vi "WaitButtonPress.vi"(8 "error in":errorcluster, 11 "GlobalDataRef":refnum<data-value>) -> (0 "error out":errorcluster, 1 "Timed Out":bool, 2 "Short=1, (Long=0)Press":bool, 3 "GlobalDataRef":refnum<data-value>)   [LabVIEW 2015]
uses:
  ProjectFiles/TypeDefs/GlobalData.ctl
  Telegram/Methods/TypeDefs/ReplyKeyboardMarkup.ctl
  <vilib>/Utility/error.llb/Error Cluster From Error Code.vi
  <vilib>/RVI Host/nirviSupport.llb/nirviErrorClusterFromErrorCode.vi
  <vilib>/rvi/errors/niLvFpgaAdjustHostInterfaceError.vi
  <vilib>/rvi/interface/nirviMethod/nirviMethod.xnode
  <vilib>/rvi/interface/nirviReadWriteControl/nirviReadWriteControl.xnode
  <vilib>/rvi/interface/nirviMethod/StockFPGA_InlinedMethodWaitForSingleIRQ.vi
  <vilib>/FPGAPlugInAG/Dynamic/niLvFpga_WaitOnIrq_Dynamic.vi
  <vilib>/FPGAPlugInAG/Dynamic/niLvFpga_AcknowledgeIrq_Dynamic.vi
  NiFpgaLv.dll
  <vilib>/rvi/interface/Simulation/niFpgaSimulationCallBeginRW.vi
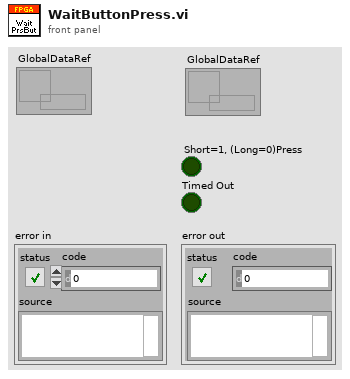
[diagram p1: front panel]
types:
  T1 = typedef "GlobalData.ctl" = cluster{"FPGA VI Ref":refnum<k20>, "Token":string, "ActiveChats":cluster{"ChatId":i32, "Type":string}[], "ActiveKeyboards":cluster{"Chat#":i32, "ReplyKeyboardMarkup":T2}[], "RefStringIn":refnum<vi>}
  T2 = typedef "ReplyKeyboardMarkup.ctl" = cluster{"keyboard":cluster{"text":string, "req_loc":bool}[][], "resize_keyboard":bool, "one_time_keyboard":bool, "selective":bool}
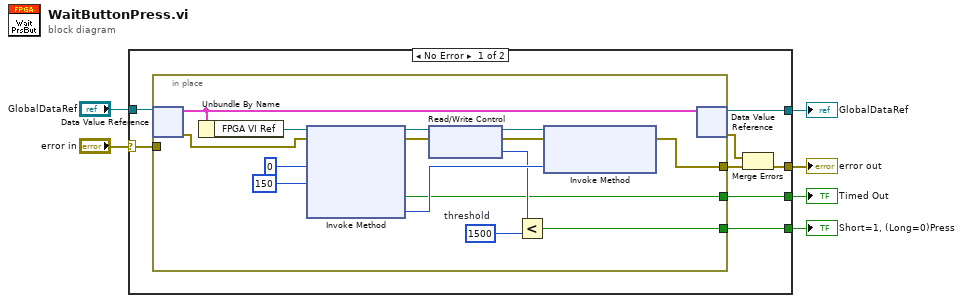
[diagram p0: block diagram]
diagram:
  n1 = case shown="No Error" "error in" {
    selector: "error in" -> [w13 w31]
    tunnel: "GlobalDataRef" -> [w14 w30]
    tunnel: [w12 _] -> w4
    tunnel: [w11 _] -> w3
    tunnel: [w7 w31] -> w2
    tunnel: [w10 w30] -> w1
    frame No Error {
      n2 = in-place {
        in-place-border: w13 -> [_]
        in-place-border: [w18] -> w9
        in-place-border: [w16] -> w12
        in-place-border: [w15] -> w11
        w20 = i16 1500  # threshold
        n3 = in-place-dvr #1(w14) -> (w29:T1, w17:errorcluster)
        n4 = Unbundle By Name(w29) -> ("FPGA VI Ref"=w19:refnum<k20>)
        n5 = xnode "Invoke Method"("FPGA VI Reference In"=w19, "error in"=w17, "IRQ Number(s)"=0, "Timeout (ms)"=150) -> ("FPGA VI Reference Out"=w25:refnum<k20>, "error out"=w26:errorcluster, "Timed Out"=w16:bool, "IRQ(s) Asserted"=w23:i32)
        n6 = xnode "Read/Write Control"("FPGA VI Reference In"=w25, "error in"=w26) -> ("FPGA VI Reference Out"=w28:refnum<k20>, "error out"=w27:errorcluster, "Duration 2"=w21:i16)
        n7 = Less?(x=w21, y=w20) -> (x < y?=w15:bool)
        n8 = xnode "Invoke Method"("FPGA VI Reference In"=w28, "error in"=w27, "IRQ Number(s)"=w23) -> ("error out"=w18:errorcluster)  [unwired: 1 out]
        n9 = in-place-dvr #1(w29) -> (w10:refnum<data-value>, w8:errorcluster)
      }
      n10 = Merge Errors(w8, w9) -> (w7:errorcluster)
    }
    frame Error {
    }
  }
  "error out" <- w2
  "Short=1, (Long=0)Press" <- w3
  "Timed Out" <- w4
  "GlobalDataRef" <- w1
